vi "TDM2TDMSCheckPaths.vi"(8 "error in (no error)":errorcluster, 10 "TDM Path In":path=path "C:/Documents and Settings/jslocum/Desktop/Projects/TDM_TDMS/Files/WriteAllChannelTypes.TDM", 11 "New TDMS Path In":path=path "C:/Documents and Settings/jslocum/Desktop/Projects/TDM_TDMS/Files/written files/TDM_With_Details_NEW.tdms") -> (0 "error out":errorcluster, 2 "TDM File Out":path, 3 "TDMS File Out":path)   [LabVIEW 2020]
doc: "This VI checks to see if valid paths have been entered for the source and target files. If not, a dialog prompts for a valid file path. If only a directory is given for the target path, then a default filename is created in that directory using the source filename and the target extension."
uses:
  <vilib>/Utility/tdmsutil.llb/TDMSFileViewerLocalizedText.vi
  Instance           1 26Saved   TDM2TDMSCheckPaths .vi
  Instance           2 26Saved   TDM2TDMSCheckPaths .vi
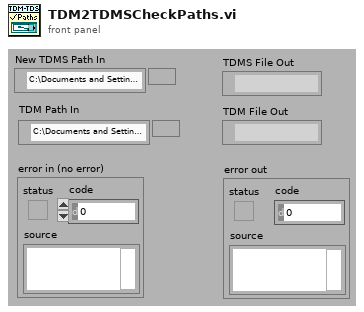
[diagram p1: front panel]
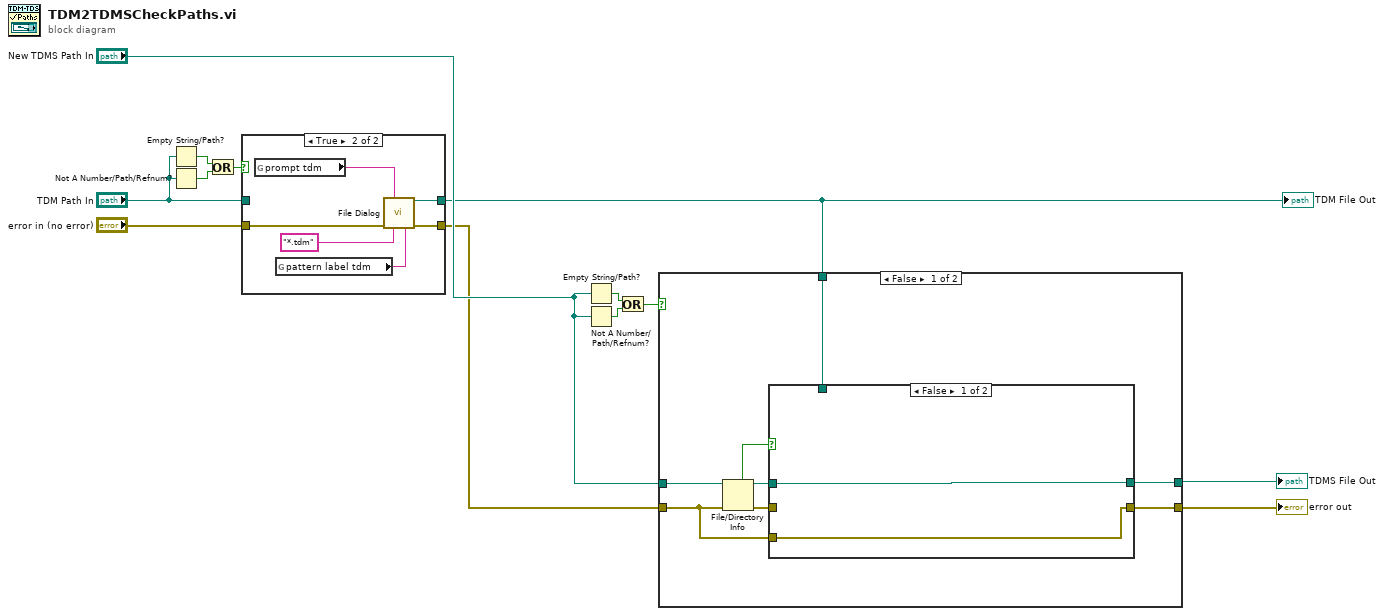
[diagram p0: block diagram]
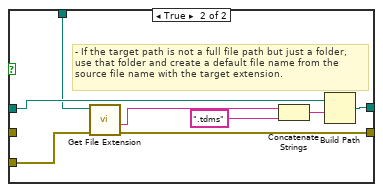
[diagram p2: hidden frame]
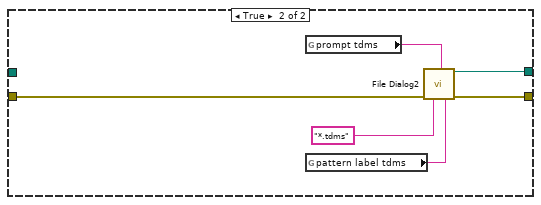
[diagram p3: hidden frame]
diagram:
  n1 = Empty String/Path?(string/path="TDM Path In") -> (empty?=w11:bool)
  n2 = Not A Number/Path/Refnum?(number/path/refnum="TDM Path In") -> (NaN/Path/Refnum?=w10:bool)
  n3 = Or(x=w11, y=w10) -> (x .or. y?=w9:bool)
  n4 = case shown="True" w9 {
    tunnel: "TDM Path In" -> [w15 _]
    tunnel: [w15 w21] -> w3
    tunnel: [w14 w20] -> w4
    tunnel: "error in (no error)" -> [w14 w19]
    frame False {
    }
    frame True {
      n5 = global read "TDMSFileViewerLocalizedText.vi" "prompt tdm"() -> (w18:string)
      n6 = global read "TDMSFileViewerLocalizedText.vi" "pattern label tdm"() -> (w17:string)
      n7 = call "File Dialog"("prompt"=w18, "error in"=w19, "pattern (all files)"="*.tdm" ("pattern label"), "pattern label"=w17) -> ("selected path"=w21:path, "error out"=w20:errorcluster)  [unwired: 8 in, 2 out]
    }
  }
  "TDM File Out" <- w3
  n8 = Empty String/Path?(string/path="New TDMS Path In") -> (empty?=w6:bool)
  n9 = Not A Number/Path/Refnum?(number/path/refnum="New TDMS Path In") -> (NaN/Path/Refnum?=w7:bool)
  n10 = Or(x=w6, y=w7) -> (x .or. y?=w8:bool)
  n11 = case shown="False" w8 {
    tunnel: "New TDMS Path In" -> [w26 _]
    tunnel: w4 -> [w23 w42]
    tunnel: [w25 w43] -> w1
    tunnel: [w24 w44] -> w2
    tunnel: w3 -> [w22 _]
    frame False {
      n12 = File/Directory Info(path=w26, error in=w23) -> (path out=w28:path, directory=w27:bool, error out=w29:errorcluster)  [unwired: 4 out]
      n13 = case shown="False" w27 {
        tunnel: [w31 w37] -> w24
        tunnel: w28 -> [w31 w38]
        tunnel: w23 -> [w30 w39]
        tunnel: [w30 w36] -> w25
        tunnel: w29 -> [_ _]
        tunnel: w22 -> [_ w32]
        frame False {
        }
        frame True {
          # "- If the target path is not a full file path but just a folder,\nuse that folder and create a default file name from the\nsource file name with the target extension."
          n14 = call <vilib>:"Get File Extension.vi"("error in (no error)"=w39, "file"=w32) -> ("error out"=w36:errorcluster, "filename without extension"=w35:string)  [unwired: 5 in, 3 out]
          n15 = Concatenate Strings(w35, ".tdms") -> (w34:string)
          n16 = Build Path(base path=w38, name or relative path=w34) -> (appended path=w37:path)
        }
      }
    }
    frame True {
      n17 = global read "TDMSFileViewerLocalizedText.vi" "prompt tdms"() -> (w45:string)
      n18 = global read "TDMSFileViewerLocalizedText.vi" "pattern label tdms"() -> (w40:string)
      n19 = call "File Dialog2"("prompt"=w45, "error in"=w42, "pattern (all files)"="*.tdms" ("pattern label"), "pattern label"=w40) -> ("selected path"=w44:path, "error out"=w43:errorcluster)  [unwired: 8 in, 2 out]
    }
  }
  "error out" <- w1
  "TDMS File Out" <- w2
